vi "LUT - Test Setter.vi"(8 "error in (no error)":errorcluster) -> (0 "error out":errorcluster)   [LabVIEW 2017]
uses:
  <vilib>/addons/_JKI Toolkits/Caraya/classes/Assert/Assert True.vi
  <vilib>/addons/_JKI Toolkits/Caraya/classes/Assert/Assert Equal Value and Type_Variant.vi
  <vilib>/addons/_JKI Toolkits/Caraya/classes/Test/Test.lvclass
  <vilib>/addons/_JKI Toolkits/Caraya/classes/Assert/Assert.lvclass
  src/LUT/LUT.lvclass
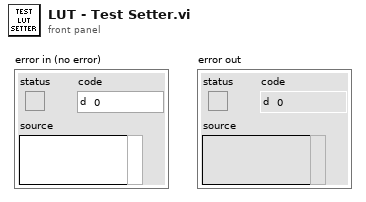
[diagram p1: front panel]
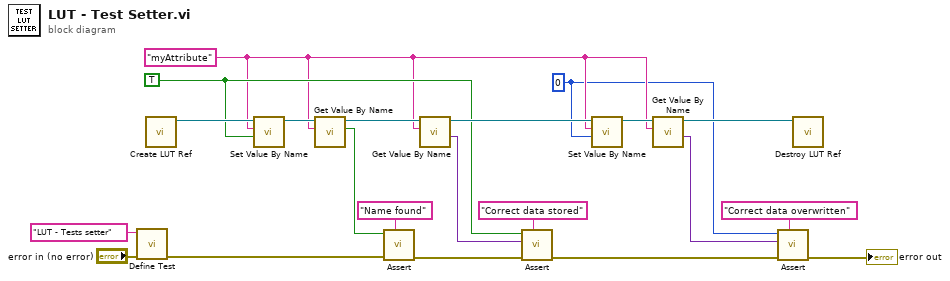
[diagram p0: block diagram]
diagram:
  w1 = 0
  w7 = TRUE
  w6 = "myAttribute"
  n1 = call <vilib>:"Define Test.vi"("error in (no error)"="error in (no error)", "Label (VI Title)"="LUT - Tests setter") -> ("error out"=w21:errorcluster)  [unwired: 9 in]
  n2 = call "Create LUT Ref.vi"() -> ("LUT out"=w18:refnum<class "LUT.lvclass">)  [unwired: 10 in, 1 out]
  n3 = call "Set Value By Name.vi"("Value"=w7, "Name"=w6, "LUT in"=w18) -> ("LUT out"=w17:refnum<class "LUT.lvclass">)  [unwired: 6 in, 2 out]
  n4 = call "Get Value By Name.vi"("Name"=w6, "LUT in"=w17) -> ("found?"=w15:bool, "LUT out"=w14:refnum<class "LUT.lvclass">)  [unwired: 6 in, 2 out]
  n5 = call-poly <vilib>:"Assert.vi"("Label"="Name found", "error in (no error)"=w21, "True?"=w15) -> ("error out"=w12:errorcluster)  [unwired: 8 in]
  n6 = call "Get Value By Name.vi"("Name"=w6, "LUT in"=w14) -> ("Value"=w11:variant, "LUT out"=w9:refnum<class "LUT.lvclass">)  [unwired: 6 in, 2 out]
  n7 = call-poly <vilib>:"Assert.vi"("Label"="Correct data stored", "error in (no error)"=w12, "Y"=w11, "X"=w7) -> ("error out"=w4:errorcluster)  [unwired: 7 in]
  n8 = call "Set Value By Name.vi"("Value"=w1, "Name"=w6, "LUT in"=w9) -> ("LUT out"=w10:refnum<class "LUT.lvclass">)  [unwired: 6 in, 2 out]
  n9 = call "Get Value By Name.vi"("Name"=w6, "LUT in"=w10) -> ("Value"=w2:variant, "LUT out"=w8:refnum<class "LUT.lvclass">)  [unwired: 6 in, 2 out]
  n10 = call-poly <vilib>:"Assert.vi"("Label"="Correct data overwritten", "error in (no error)"=w4, "Y"=w2, "X"=w1) -> ("error out"=→"error out":errorcluster)  [unwired: 7 in]
  n11 = call "Destroy LUT Ref.vi"("LUT in"=w8) -> ()  [unwired: 10 in, 1 out]
